vi "serial_demux.vi"() -> ()   [LabVIEW 2012]
doc: "Each output represents one bit of the output word, which, in 74 series counter ICs is usually 4 bits long, and the size of the output word depends on the number of flip-flops that make up the counter. The output lines of a 4-bit counter represent the values 20, 21, 22 and 23, or 1,2,4 and 8 respectively. They are normally shown in schematic diagrams in reverse order, with the least significant bit at the left, this is to enable the schematic diagram to show the circuit following the convention that signals flow from left to right, therefore in this case the CK input is at the left."
panel:
  out "Computed voltage 1":dbl
  out "Computed Voltage 2":dbl
  out "bit16":dbl
  out "bit15":dbl
  out "bit14":dbl
  out "bit12":dbl
  out "bit13":dbl
  out "bit11":dbl
  out "bit10":dbl
  out "bit9":dbl
  out "Digital 2":dbl
  out "Count":u32
  out "bit8":dbl
  out "bit7":dbl
  out "bit6":dbl
  out "bit5":dbl
  out "bit4":dbl
  out "bit3":dbl
  out "bit2":dbl
  out "bit1":dbl
  out "Digital 1":sgl
  out "Bit3":bool
  in  "Stop":bool
  out "Bit0":bool
  out "Bit1":bool
  out "Bit2":bool
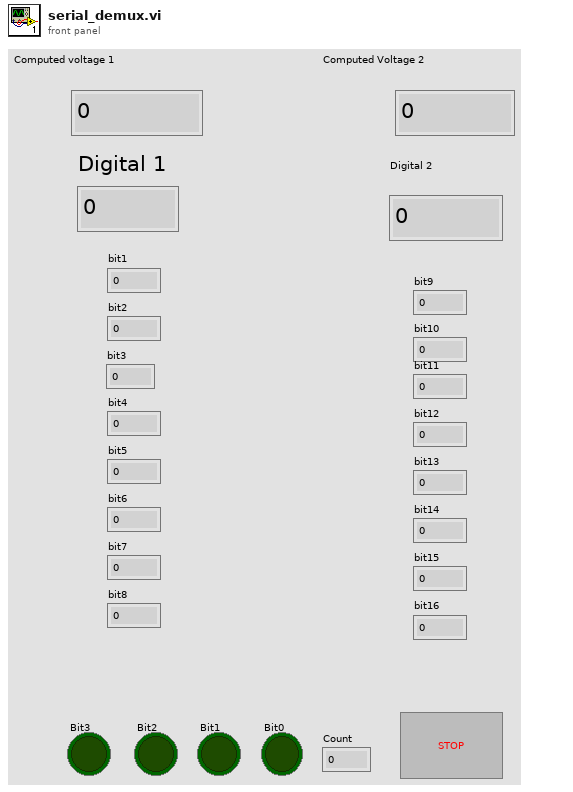
[diagram p1: front panel]
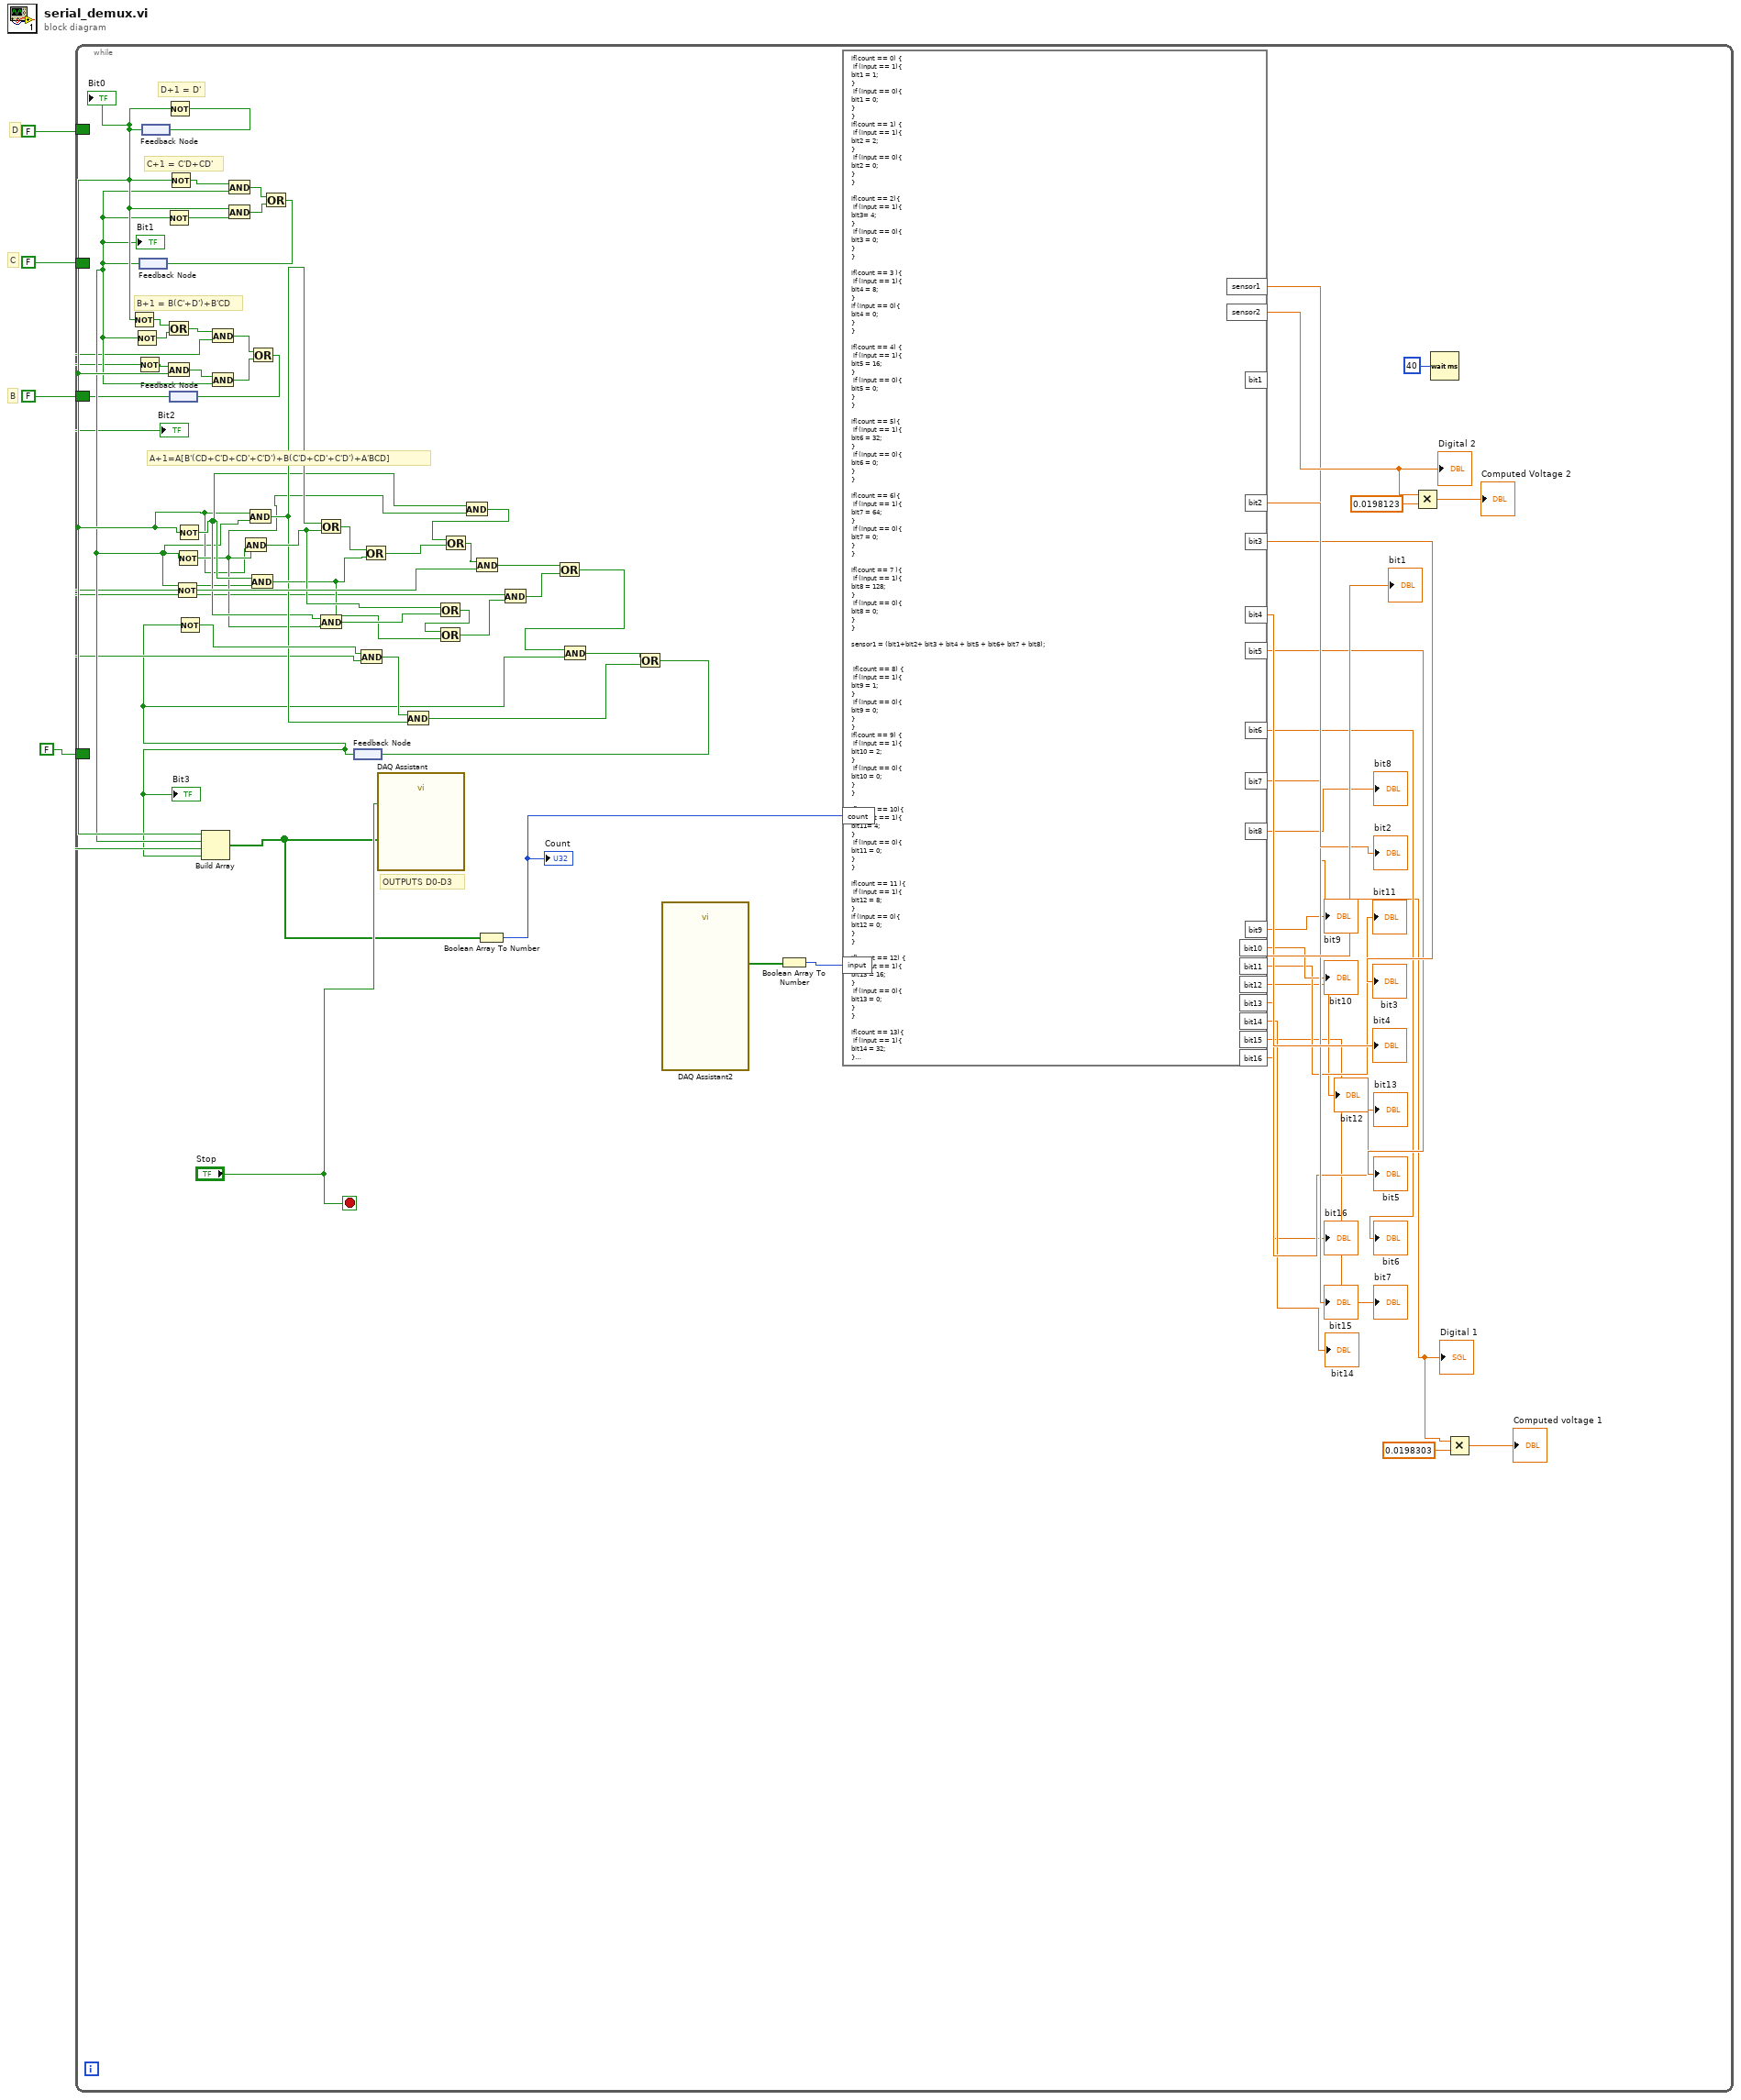
[diagram p0: block diagram]
diagram:
  # "D"
  # "C"
  # "B"
  n1 = while {
    border: FALSE -> [_]
    border: FALSE -> [_]
    border: FALSE -> [_]
    border: FALSE -> [_]
    stop <- "Stop" stop-if-true
    # "OUTPUTS D0-D3"
    # "A+1=A[B'(CD+C'D+CD'+C'D')+B(C'D+CD'+C'D')+A'BCD]"
    # "D+1 = D'"
    # "C+1 = C'D+CD'"
    # "B+1 = B(C'+D')+B'CD"
    n2 = feedback #1() -> (w32:bool)
    "Bit1" <- w32
    n3 = Not(x=w32) -> (.not. x?=w38:bool)
    n4 = feedback #2() -> (w33:bool)
    "Bit0" <- w33
    n5 = Not(x=w33) -> (.not. x?=w65:bool)
    n6 = Not(x=w32) -> (.not. x?=w66:bool)
    n7 = Or(x=w65, y=w38) -> (x .or. y?=w39:bool)
    n8 = Not(x=w33) -> (.not. x?=w71:bool)
    n9 = feedback-in #2(w71) -> ()
    n10 = Not(x=w33) -> (.not. x?=w67:bool)
    n11 = feedback #3() -> (w31:bool)
    "Bit2" <- w31
    n12 = Not(x=w31) -> (.not. x?=w37:bool)
    n13 = And(x=w37, y=w33) -> (x .and. y?=w63:bool)
    n14 = Not(x=w31) -> (.not. x?=w60:bool)
    n15 = Not(x=w32) -> (.not. x?=w43:bool)
    n16 = Not(x=w33) -> (.not. x?=w44:bool)
    n17 = And(x=w39, y=w31) -> (x .and. y?=w64:bool)
    n18 = And(x=w63, y=w32) -> (x .and. y?=w62:bool)
    n19 = And(x=w67, y=w32) -> (x .and. y?=w69:bool)
    n20 = And(x=w33, y=w66) -> (x .and. y?=w70:bool)
    n21 = And(x=w43, y=w33) -> (x .and. y?=w53:bool)
    n22 = And(x=w33, y=w32) -> (x .and. y?=w48:bool)
    n23 = And(x=w44, y=w32) -> (x .and. y?=w52:bool)
    n24 = Or(x=w64, y=w62) -> (x .or. y?=w61:bool)
    n25 = feedback-in #3(w61) -> ()
    n26 = Or(x=w69, y=w70) -> (x .or. y?=w68:bool)
    n27 = feedback-in #1(w68) -> ()
    n28 = Or(x=w48, y=w53) -> (x .or. y?=w54:bool)
    n29 = And(x=w44, y=w43) -> (x .and. y?=w59:bool)
    n30 = feedback #4() -> (w30:bool)
    "Bit3" <- w30
    n31 = Not(x=w30) -> (.not. x?=w55:bool)
    n32 = Build Array(w33, w32, w31, w30) -> (w20:bool[])
    n33 = And(x=w55, y=w31) -> (x .and. y?=w49:bool)
    n34 = Or(x=w54, y=w52) -> (x .or. y?=w41:bool)
    n35 = call "DAQ Assistant"("data"=w20, "stop (T)"="Stop") -> ()  [unwired: 16 in, 2 out]
    n36 = And(x=w49, y=w48) -> (x .and. y?=w46:bool)
    n37 = Or(x=w53, y=w59) -> (x .or. y?=w51:bool)
    n38 = Or(x=w51, y=w52) -> (x .or. y?=w50:bool)
    n39 = And(x=w44, y=w43) -> (x .and. y?=w42:bool)
    n40 = Or(x=w42, y=w41) -> (x .or. y?=w40:bool)
    n41 = And(x=w40, y=w60) -> (x .and. y?=w58:bool)
    n42 = Boolean Array To Number(Boolean array=w20) -> (number=w19:u32)
    "Count" <- w19
    n43 = And(x=w31, y=w50) -> (x .and. y?=w57:bool)
    n44 = Or(x=w58, y=w57) -> (x .or. y?=w56:bool)
    n45 = And(x=w56, y=w30) -> (x .and. y?=w47:bool)
    n46 = Or(x=w47, y=w46) -> (x .or. y?=w45:bool)
    n47 = feedback-in #4(w45) -> ()
    n48 = call "DAQ Assistant2"() -> ("data"=w35:bool[])  [unwired: 17 in, 2 out]
    n49 = Boolean Array To Number(Boolean array=w35) -> (number=w36:u32)
    n50 = formula code="if(count == 0) {\n if (input == 1){\nbit1 = 1;\n}\n if (input == 0){\nbit1 = 0;\n}\n}\nif(count == 1) {\n if (input == 1){\nbit2 = 2;\n}\n if (input == 0){\nbit2 = 0;\n}\n}\n\nif(count == 2){\n if (input == 1){\nbit3= 4;\n}\n if (input == 0){\nbit3 = 0;\n}\n}\n\nif(count == 3 ){\n if (input == 1){\nbit4 = 8;\n}\nif (input == 0){\nbit4 = 0;\n}\n}\n\nif(count == 4) {\n if (input == 1){\nbit5 = 16;\n}\n if (input == 0){\nbit5 = 0;\n}\n}\n\nif(count == 5){\n if (input == 1){\nbit6 = 32;\n}\n if (input == 0){\nbit6 = 0;\n}\n}\n\nif(count == 6){\n if (input == 1){\nbit7 = 64;\n}\n if (input == 0){\nbit7 = 0;\n}\n}\n\nif(count == 7 ){\n if (input == 1){\nbit8 = 128;\n}\n if (input == 0){\nbit8 = 0;\n}\n}\n\nsensor1 = (bit1+bit2+ bit3 + bit4 + bit5 + bit6+ bit7 + bit8);\n\n\n if(count == 8) {\n if (input == 1){\nbit9 = 1;\n}\n if (input == 0){\nbit9 = 0;\n}\n}\nif(count == 9) {\n if (input == 1){\nbit10 = 2;\n}\n if (input == 0){\nbit10 = 0;\n}\n}\n\nif(count == 10){\n if (input == 1){\nbit11= 4;\n}\n if (input == 0){\nbit11 = 0;\n}\n}\n\nif(count == 11 ){\n if (input == 1){\nbit12 = 8;\n}\nif (input == 0){\nbit12 = 0;\n}\n}\n\nif(count == 12) {\n if (input == 1){\nbit13 = 16;\n}\n if (input == 0){\nbit13 = 0;\n}\n}\n\nif(count == 13){\n if (input == 1){\nbit14 = 32;\n}\n if (input == 0){\nbit14 = 0;\n}\n}\n\nif(count == 14){\n if (input == 1){\nbit15 = 64;\n}\n if (input == 0){\nbit15 = 0;\n}\n}\n\nif(count == 15 ){\n if (input == 1){\nbit16 = 128;\n}\n if (input == 0){\nbit16 = 0;\n}\n}\n\nsensor2 = (bit9+bit15+ bit10 + bit11 + bit12 + bit13+ bit14 + bit16);"("count"=w19, "input"=w36) -> ("sensor1"=w5:dbl, "bit1"=→"bit1":dbl, "bit2"=→"bit2":dbl, "bit3"=→"bit3":dbl, "bit4"=→"bit4":dbl, "bit5"=→"bit5":dbl, "bit6"=→"bit6":dbl, "bit7"=→"bit7":dbl, "bit8"=→"bit8":dbl, "bit9"=→"bit9":dbl, "bit10"=→"bit10":dbl, "bit11"=→"bit11":dbl, "bit13"=→"bit13":dbl, "bit14"=→"bit14":dbl, "bit15"=→"bit15":dbl, "bit16"=→"bit16":dbl, "bit12"=→"bit12":dbl, "sensor2"=w10:dbl)
    "Digital 1" <- w5
    "Digital 2" <- w10
    n51 = Multiply(x=w10, y=0.0198123) -> (x*y=→"Computed Voltage 2":dbl)
    n52 = Wait (ms)(milliseconds to wait=u32 40) -> ()  [unwired: 1 out]
    n53 = Multiply(x=w5, y=0.0198303) -> (x*y=→"Computed voltage 1":dbl)
  }
